vi "SaveFeedForwardFile.vi"(8 "error in":errorcluster, 9 "values Q":dbl[](array[numeric]), 10 "values I":dbl[](array[numeric]), 11 "Path":path) -> (0 "error out":errorcluster)   [LabVIEW 2018]
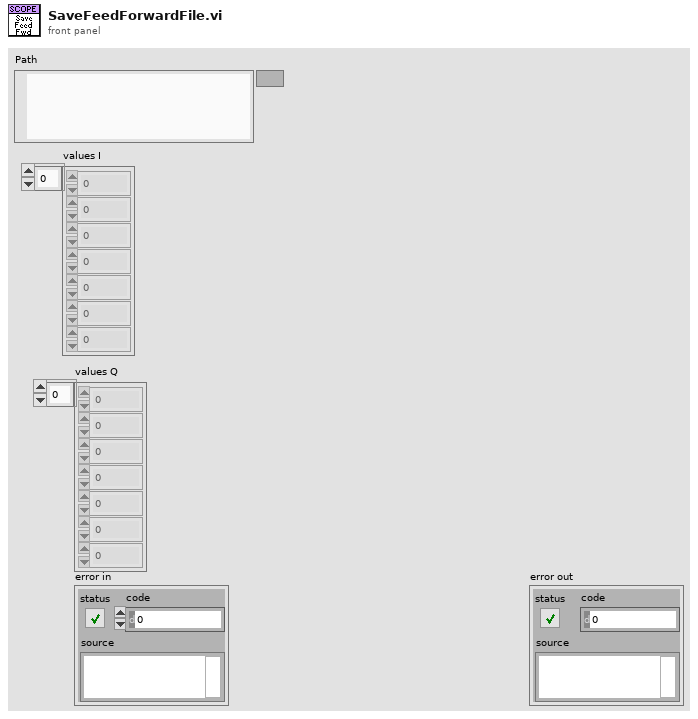
[diagram p1: front panel]
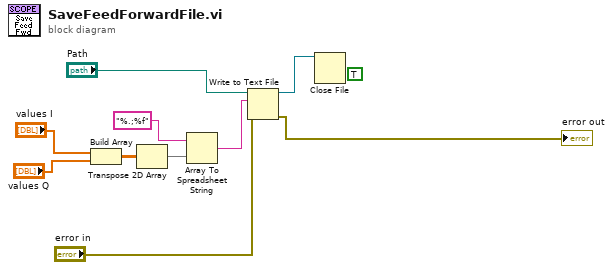
[diagram p0: block diagram]
diagram:
  (unwired) TRUE ("replace all? (F)")
  n1 = Build Array("values I", "values Q") -> (w5:dbl[][])
  n2 = Transpose 2D Array(2D array=w5) -> (transposed array=w1:dbl[][])
  n3 = Array To Spreadsheet String(array=w1, 3:"%.;%f" ("format string")) -> (spreadsheet string=w3:string)  [unwired: 1 in]
  n4 = Write to Text File(file (use dialog)="Path", text=w3, error in="error in") -> (refnum out=w9:refnum<file>, error out=→"error out":errorcluster)  [unwired: 1 in, 1 out]
  n5 = Close File(refnum=w9) -> ()  [unwired: 1 in, 2 out]
